vi "Close Instrument.vi"(8 "error in (no error)":errorcluster, 11 "NI Digitizer.lvclass in":refnum<class "NI Digitizer.lvclass">) -> (0 "error out":errorcluster, 3 "NI Digitizer.lvclass out":refnum<class "NI Digitizer.lvclass">)   [LabVIEW 2011, in "NI Digitizer.lvclass"]
uses:
  NI Digitizer.lvclass
  NI Digitizer.lvclass/NI Digitizer.ctl
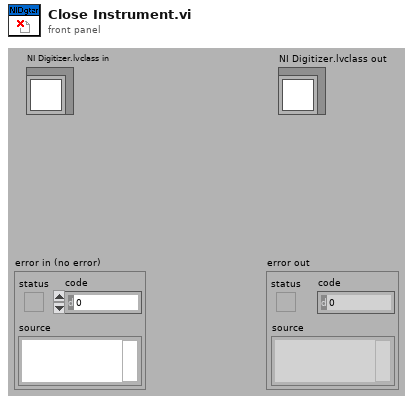
[diagram p1: front panel]
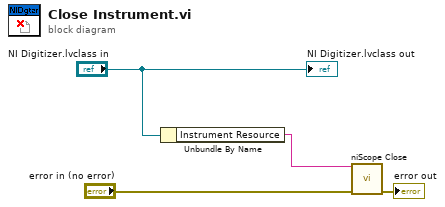
[diagram p0: block diagram]
diagram:
  n1 = Unbundle By Name("NI Digitizer.lvclass in") -> ("Instrument Resource"=w1:string)
  n2 = call <instrlib>:"niScope Close.vi"("instrument handle"=w1, "error in"="error in (no error)") -> ("error out"=→"error out":errorcluster)  [unwired: 13 out]
  "NI Digitizer.lvclass out" <- "NI Digitizer.lvclass in"
